vi "Red Button.vi"() -> ()   [LabVIEW 2020]
uses:
  Red Button Enum.ctl
panel:
  in  "Switch":bool
  out "State":T1
  in  "stop":bool
  in  "1":bool
  in  "2":bool
  in  "3":bool
  out "Lamp":bool
  in  "Check for every step":bool
  # "The password is \"1-2-3\" consequtively, you should push \"check for every step\"in each step\nafter you select the password. Then turn on the switch and then press \"check for every step\"\n again. You can easily change the password by giving desiredboolean values inside case\n structure in the 1,2,3 cases, in the block diagram."
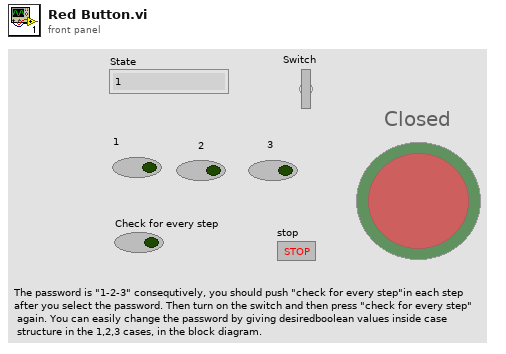
[diagram p1: front panel]
types:
  T1 = typedef "Red Button Enum.ctl" = enum16{"1", "2", "3", "Unlocked", "Open"}
  T2 = enum8{"Enabled", "Disabled", "Disabled and Grayed Out"}
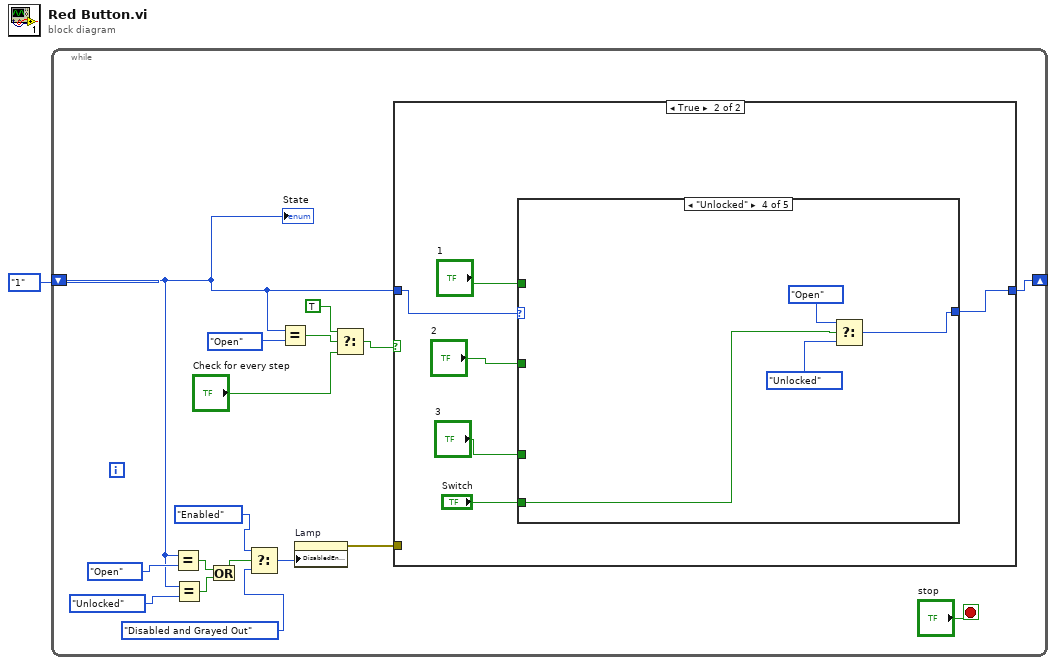
[diagram p0: block diagram]
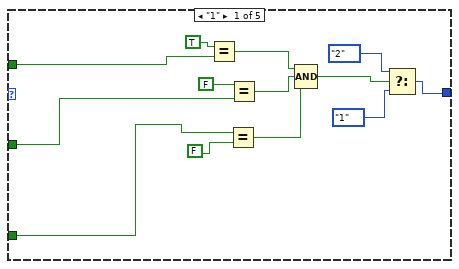
[diagram p3: hidden frame]
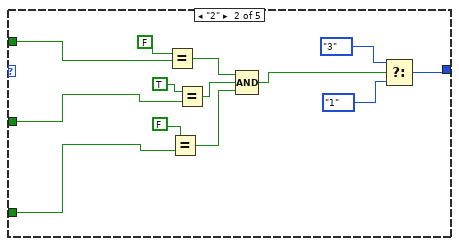
[diagram p4: hidden frame]
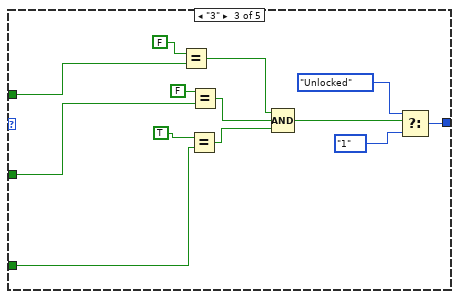
[diagram p5: hidden frame]
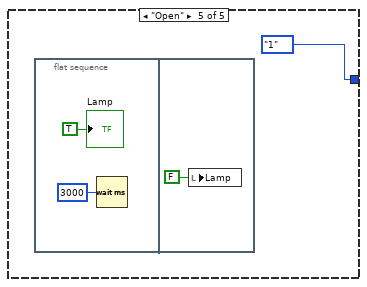
[diagram p6: hidden frame]
diagram:
  n1 = while {
    shift-right: [w17] -> _
    shift-left: Red_Button_Enum."1" ("Enum") -> [w5]
    stop <- "stop" stop-if-true
    n2 = Equal?(x=w5, y=Red_Button_Enum."Open" ("Enum")) -> (x = y?=w4:bool)
    n3 = Equal?(x=w5, y=Red_Button_Enum."Unlocked" ("Enum")) -> (x = y?=w3:bool)
    n4 = Or(x=w4, y=w3) -> (x .or. y?=w2:bool)
    n5 = Select(t=T2."Enabled" ("Disabled"), s=w2, f=T2."Disabled and Grayed Out" ("Disabled")) -> (s? t:f=w10:T2)
    n6 = Equal?(x=w5, y=Red_Button_Enum."Open" ("Enum")) -> (x = y?=w16:bool)
    n7 = property on="Lamp" class="Bool"("DisabledEnum"=w10) -> (error out=w9:errorcluster)  [unwired: 2 in, 1 out]
    n8 = Select(t=TRUE, s=w16, f="Check for every step") -> (s? t:f=w15:bool)
    n9 = case shown="True" w15 {
      tunnel: w5 -> [w19 w21]
      tunnel: [w19 w25] -> w17
      tunnel: w9 -> [_ _]
      frame False {
      }
      frame True {
        n10 = case shown="\"Unlocked\"" w21 {
          tunnel: [w31 w51 w64 w68 Red_Button_Enum."1" ("Enum")] -> w25
          tunnel: "1" -> [w30 w43 w56 _ _]
          tunnel: "2" -> [w29 w42 w55 _ _]
          tunnel: "3" -> [w28 w41 w54 _ _]
          tunnel: "Switch" -> [_ _ _ w65 _]
          frame "1" {
            n11 = Equal?(x=TRUE, y=w30) -> (x = y?=w35:bool)
            n12 = Equal?(x=w28, y=FALSE) -> (x = y?=w33:bool)
            n13 = Equal?(x=FALSE, y=w29) -> (x = y?=w34:bool)
            n14 = Compound Arithmetic op=AND(w35, w34, w33) -> (w32:bool)
            n15 = Select(t=Red_Button_Enum."2" ("Enum"), s=w32, f=Red_Button_Enum."1" ("Enum")) -> (s? t:f=w31:T1)
          }
          frame "2" {
            n16 = Equal?(x=FALSE, y=w43) -> (x = y?=w47:bool)
            n17 = Equal?(x=FALSE, y=w41) -> (x = y?=w45:bool)
            n18 = Equal?(x=TRUE, y=w42) -> (x = y?=w46:bool)
            n19 = Compound Arithmetic op=AND(w47, w46, w45) -> (w44:bool)
            n20 = Select(t=Red_Button_Enum."3" ("Enum"), s=w44, f=Red_Button_Enum."1" ("Enum")) -> (s? t:f=w51:T1)
          }
          frame "3" {
            n21 = Equal?(x=FALSE, y=w56) -> (x = y?=w60:bool)
            n22 = Equal?(x=TRUE, y=w54) -> (x = y?=w58:bool)
            n23 = Equal?(x=FALSE, y=w55) -> (x = y?=w59:bool)
            n24 = Compound Arithmetic op=AND(w60, w59, w58) -> (w57:bool)
            n25 = Select(t=Red_Button_Enum."Unlocked" ("Enum"), s=w57, f=Red_Button_Enum."1" ("Enum")) -> (s? t:f=w64:T1)
          }
          frame "Unlocked" {
            n26 = Select(t=Red_Button_Enum."Open" ("Enum"), s=w65, f=Red_Button_Enum."Unlocked" ("Enum")) -> (s? t:f=w68:T1)
          }
          frame "Open" {
            n27 = flat-sequence {
              frame #0 {
                n28 = Wait (ms)(milliseconds to wait=u32 3000) -> ()  [unwired: 1 out]
                "Lamp" <- TRUE ("Lamp")
              }
              frame #1 {
                n29 = local write "Lamp"(FALSE ("Lamp")) -> ()
              }
            }
          }
        }
      }
    }
    "State" <- w5
  }
